vi "oef15.vi"() -> ()   [LabVIEW 2021]
panel:
  out "HowMany":dbl
  in  "Value":dbl
  in  "Array":dbl[](array[numeric])
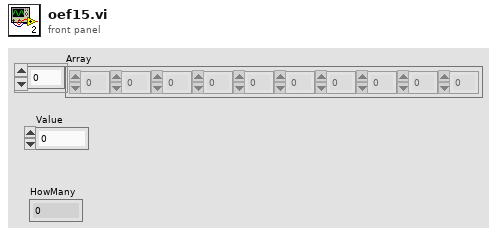
[diagram p1: front panel]
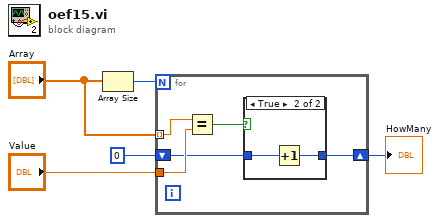
[diagram p0: block diagram]
diagram:
  n1 = Array Size(array="Array") -> (size(s)=w5:i32)
  n2 = for {
    N: w5 -> [_]
    tunnel: "Array" -> [w10] mode=indexing
    tunnel: "Value" -> [w9]
    shift-right: [w7] -> w2
    shift-left: 0 -> [w6]
    n3 = Equal?(x=w10, y=w9) -> (x = y?=w8:bool)
    n4 = case shown="True" w8 {
      tunnel: w6 -> [w11 w13]
      tunnel: [w11 w12] -> w7
      frame False {
      }
      frame True {
        n5 = Increment(x=w13) -> (x+1=w12:i32)
      }
    }
  }
  "HowMany" <- w2
